vi "Check_Reserved_Lines.vi"(8 "error in (no error)":errorcluster, 10 "Master Device in":refnum<class "Master Device.lvclass">, 11 "Pulseblaster in":refnum<class "Pulseblaster.lvclass">) -> (0 "error out":errorcluster, 2 "Master Device out":refnum<class "Master Device.lvclass">, 3 "Pulseblaster out":refnum<class "Pulseblaster.lvclass">)   [LabVIEW 2013, in "Pulseblaster.lvclass"]
uses:
  Pulseblaster.lvclass
  Master Device/Master Device.lvclass
  ColumnVIs/TriggerCol/TriggerCol.lvclass
  <vilib>/Utility/error.llb/DialogType.ctl
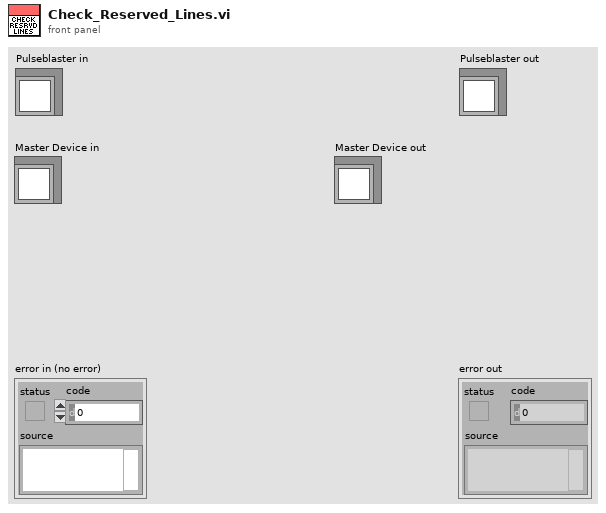
[diagram p1: front panel]
types:
  T1 = typedef "SlaveInfo.ctl" = cluster{"Triggering":bool[][], "Ramp Info":T2[], "Line Inversion":bool[], "Slaved Digital Channels":cluster{"Master Channel Number":i32, "Output States":bool[]}[]}
  T2 = typedef "RampInfo.ctl" = cluster{"Table Ramp Index":i32, "Ramp Time":dbl, "Number of Steps":i32, "Instruction Array Index":i32}
  T3 = cluster{"Master Channel Number":i32, "Output States":bool[]}[]
  T4 = typedef "DialogType.ctl" = u16
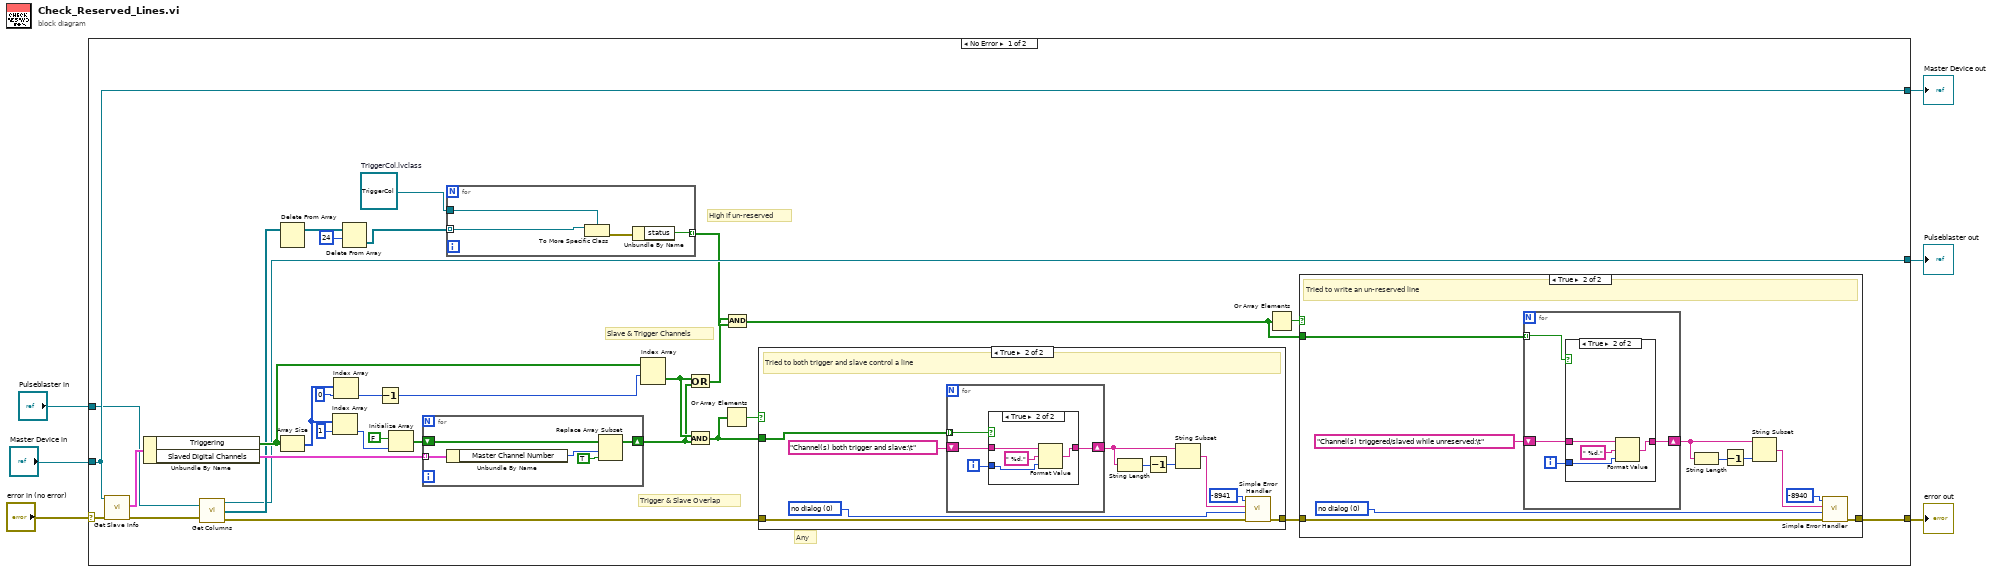
[diagram p0: block diagram]
diagram:
  n1 = case shown="No Error" "error in (no error)" {
    selector: "error in (no error)" -> [w27 w90]
    tunnel: [w23 w90] -> w5
    tunnel: [w28 w89] -> w3
    tunnel: "Pulseblaster in" -> [w29 w89]
    tunnel: "Master Device in" -> [w34 w88]
    tunnel: [w34 w88] -> w1
    frame No Error {
      w30 = refnum<class "TriggerCol.lvclass"> refnum  # TriggerCol.lvclass
      # "Slave & Trigger Channels"
      # "Trigger & Slave Overlap"
      # "High if un-reserved"
      # "Any"
      n2 = call-dynamic "Get Slave Info.vi"("error in (no error)"=w27, "Master Device in"=w34) -> ("error out"=w26:errorcluster, "Slave Info"=w38:T1)  [unwired: 7 in, 1 out]
      n3 = Unbundle By Name(w38) -> ("Triggering"=w37:bool[][], "Slaved Digital Channels"=w35:T3)
      n4 = call-dynamic "Get Columns.vi"("Device in"=w29, "error in (no error)"=w26) -> ("Device out"=w28:refnum<class "Pulseblaster.lvclass">, "Columns"=w33:refnum<class "Column.lvclass">[], "error out"=w14:errorcluster)
      n5 = Delete From Array(array=w33) -> (array with subset deleted=w32:refnum<class "Column.lvclass">[])  [unwired: 2 in, 1 out]
      n6 = Array Size(array=w37) -> (size(s)=w9:i32[])
      n7 = Index Array(array=w9, index=1) -> (element=w7:i32)
      n8 = Index Array(array=w9, index=0) -> (element=w21:i32)
      n9 = Delete From Array(array=w32, length=24) -> (deleted portion=w11:refnum<class "Column.lvclass">[])  [unwired: 1 in, 1 out]
      n10 = Decrement(x=w21) -> (x-1=w10:i32)
      n11 = Initialize Array(FALSE, w7) -> (w19:bool[])
      n12 = for {
        shift-right: [w85] -> w17
        shift-left: w19 -> [w87]
        tunnel: w35 -> [w84] mode=indexing
        n13 = Unbundle By Name(w84) -> ("Master Channel Number"=w83:i32)
        n14 = Replace Array Subset(array=w87, new element=TRUE, index=w83) -> (w85:bool[])
      }
      n15 = for {
        tunnel: w11 -> [w82] mode=indexing
        tunnel: w30 -> [w81]
        tunnel: [w79] -> w25 mode=indexing
        n16 = To More Specific Class(target class=w81, reference=w82) -> (error out=w80:errorcluster)  [unwired: 1 in, 1 out]
        n17 = Unbundle By Name(w80) -> ("status"=w79:bool)
      }
      n18 = Index Array(array=w37, index (row)=w10) -> (element=w18:bool[])  [unwired: 1 in]
      n19 = Compound Arithmetic op=OR(w18, w17) -> (w16:bool[])
      n20 = Compound Arithmetic op=AND(w18, w17) -> (w12:bool[])
      n21 = Or Array Elements(Boolean array=w12) -> (logical OR=w15:bool)
      n22 = Compound Arithmetic op=AND(w16, w25) -> (w22:bool[])
      n23 = case shown="True" w15 {
        tunnel: w14 -> [w39 w44]
        tunnel: w12 -> [_ w49]
        tunnel: [w39 w40] -> w13
        frame False {
          # "No problems"
        }
        frame True {
          w42 = T4 0 items=["no dialog", "OK message", "continue or stop message", "OK message + warnings", "continue/stop + warnings"] ("type of dialog (OK msg:1)")
          # "Tried to both trigger and slave control a line"
          n24 = for {
            tunnel: w49 -> [w53] mode=indexing
            shift-right: [w51] -> w47
            shift-left: "Channel(s) both trigger and slave:\t" -> [w52]
            i -> [w50]
            n25 = case shown="True" w53 {
              tunnel: w52 -> [w54 w58]
              tunnel: [w54 w55] -> w51
              tunnel: w50 -> [_ w56]
              frame False {
              }
              frame True {
                n26 = Format Value(string ("")=w58, format string=" %d,", value (0)=w56) -> (output string=w55:string)
              }
            }
          }
          n27 = String Length(string=w47) -> (length=w46:i32)
          n28 = Decrement(x=w46) -> (x-1=w45:i32)
          n29 = String Subset(string=w47, length (rest)=w45) -> (substring=w43:string)  [unwired: 1 in]
          n30 = call <vilib>:"Simple Error Handler.vi"("error code (no error:0)"=-8941, "error source (\" \")"=w43, "type of dialog (OK msg:1)"=w42, "error in (no error)"=w44) -> ("error out"=w40:errorcluster)  [unwired: 1 in, 4 out]
        }
      }
      n31 = Or Array Elements(Boolean array=w22) -> (logical OR=w24:bool)
      n32 = case shown="True" w24 {
        tunnel: w13 -> [w59 w63]
        tunnel: [w59 w64] -> w23
        tunnel: w22 -> [_ w69]
        frame False {
          # "No problems"
        }
        frame True {
          w61 = T4 0 items=["no dialog", "OK message", "continue or stop message", "OK message + warnings", "continue/stop + warnings"] ("type of dialog (OK msg:1)")
          # "Tried to write an un-reserved line"
          n33 = for {
            tunnel: w69 -> [w73] mode=indexing
            shift-right: [w71] -> w67
            shift-left: "Channel(s) triggered/slaved while unreserved:\t" -> [w72]
            i -> [w70]
            n34 = case shown="True" w73 {
              tunnel: w72 -> [w74 w78]
              tunnel: [w74 w75] -> w71
              tunnel: w70 -> [_ w76]
              frame False {
              }
              frame True {
                n35 = Format Value(string ("")=w78, format string=" %d,", value (0)=w76) -> (output string=w75:string)
              }
            }
          }
          n36 = String Length(string=w67) -> (length=w66:i32)
          n37 = Decrement(x=w66) -> (x-1=w65:i32)
          n38 = String Subset(string=w67, length (rest)=w65) -> (substring=w62:string)  [unwired: 1 in]
          n39 = call <vilib>:"Simple Error Handler.vi"("error code (no error:0)"=-8940, "error source (\" \")"=w62, "type of dialog (OK msg:1)"=w61, "error in (no error)"=w63) -> ("error out"=w64:errorcluster)  [unwired: 1 in, 4 out]
        }
      }
    }
    frame Error {
    }
  }
  "error out" <- w5
  "Pulseblaster out" <- w3
  "Master Device out" <- w1
